vi "to string.vi"(8 "error in":errorcluster, 11 "Logic Sequencer configuration in":refnum<class "Logic Sequencer configuration.lvclass">) -> (0 "error out":errorcluster, 1 "data":string, 2 "version":string, 3 "Logic Sequencer configuration out":refnum<class "Logic Sequencer configuration.lvclass">)   [LabVIEW 2013, in "Logic Sequencer configuration.lvclass"]
doc: "Provides an interface for saving a module configuration to a file or other serialized data source. It is recommended that all children of this class store data in two sets--data required for its own initialization, and any data required for parent initialization--and that each implementation uses the <b>Call Parent Method</b> primitive to serialize parent information."
uses:
  Logic Sequencer configuration.lvclass
  <vilib>/NI/Tag Bus Module Framework/module configuration/TBM module configuration.lvclass
  Logic Sequencer configuration.lvclass/Logic Sequencer configuration.ctl
  <vilib>/NI/Tag Bus Module Framework/root configuration/unwrap data.vi
  current version.vi
  <vilib>/NI/Tag Bus Module Framework/root configuration/TBM configuration.lvclass
  <vilib>/NI/Tag Bus Module Framework/channel/TBM channel.lvclass
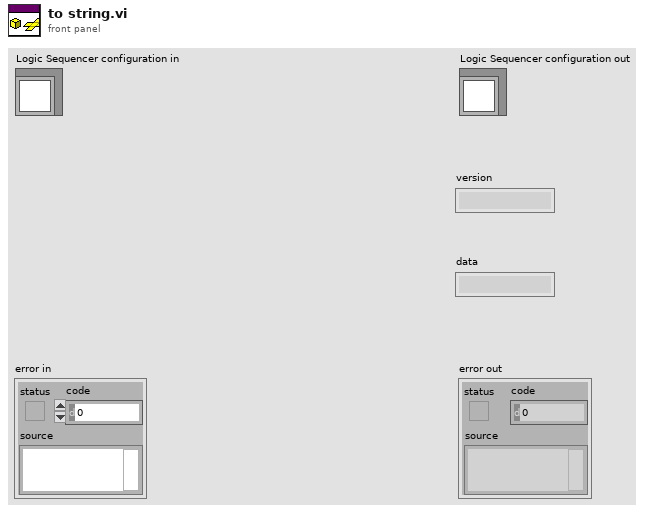
[diagram p1: front panel]
types:
  T1 = typedef "Logic Sequencer configuration.lvclass/processing channels.ctl" = cluster{"parameter":refnum<class "TBM channel.lvclass">, "result":refnum<class "TBM channel.lvclass">}
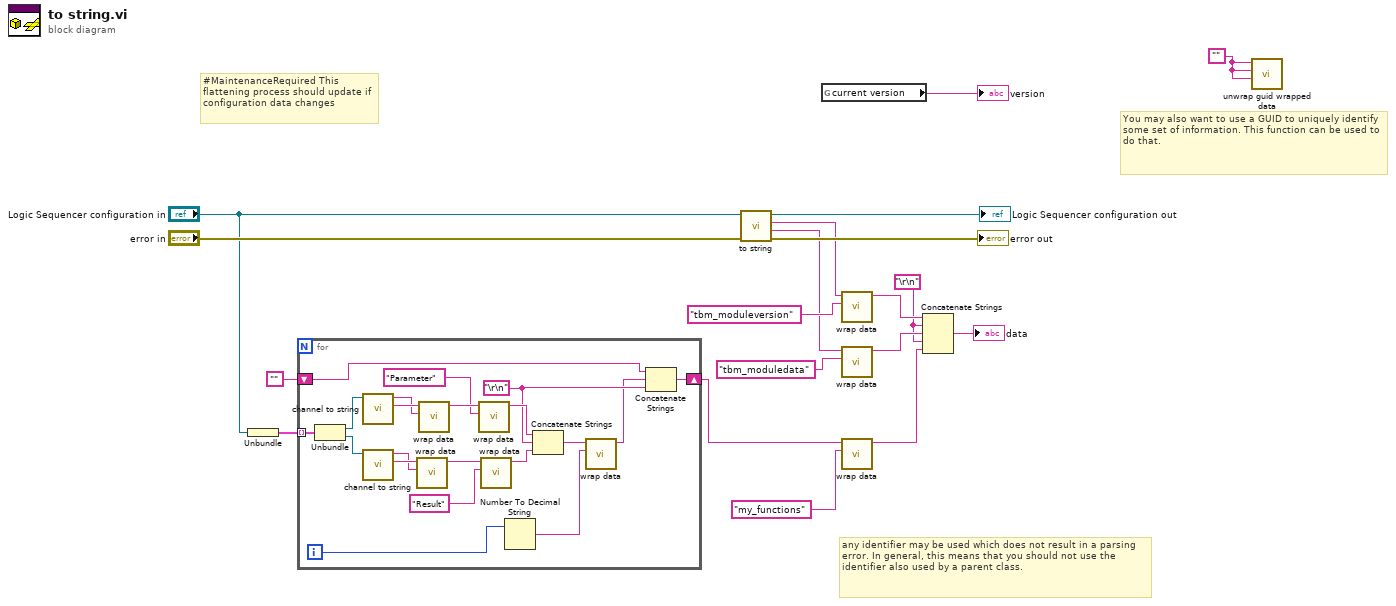
[diagram p0: block diagram]
diagram:
  w1 = "\r\n"
  w11 = ""
  # "any identifier may be used which does not result in a parsing error. In general, this means that you should not use the identifier also used by a parent class."
  # "You may also want to use a GUID to uniquely identify some set of information. This function can be used to do that."
  # "#MaintenanceRequired This flattening process should update if configuration data changes"
  n1 = Unbundle("Logic Sequencer configuration in") -> (w5:T1[])
  n2 = for {
    tunnel: w5 -> [w39] mode=indexing
    shift-right: [w26] -> w3
    shift-left: "" -> [w25]
    i -> [w23]
    w24 = "\r\n"
    n3 = Unbundle(w39) -> ("parameter"=w38:refnum<class "TBM channel.lvclass">, "result"=w37:refnum<class "TBM channel.lvclass">)
    n4 = call <vilib>:"channel to string.vi"("channel in"=w38) -> ("channel data"=w36:string, "identifier"=w33:string)  [unwired: 9 in]
    n5 = call <vilib>:"channel to string.vi"("channel in"=w37) -> ("channel data"=w35:string, "identifier"=w34:string)  [unwired: 9 in]
    n6 = call <vilib>:"wrap data.vi"("identifier"=w34, "data to wrap"=w35) -> ("wrapped data"=w30:string)  [unwired: 9 in]
    n7 = call <vilib>:"wrap data.vi"("identifier"=w33, "data to wrap"=w36) -> ("wrapped data"=w32:string)  [unwired: 9 in]
    n8 = call <vilib>:"wrap data.vi"("identifier"="Parameter", "data to wrap"=w32) -> ("wrapped data"=w28:string)  [unwired: 9 in]
    n9 = call <vilib>:"wrap data.vi"("identifier"="Result", "data to wrap"=w30) -> ("wrapped data"=w27:string)  [unwired: 9 in]
    n10 = Number To Decimal String(number=w23) -> (decimal integer string=w21:string)  [unwired: 1 in]
    n11 = Concatenate Strings(w28, w24, w27) -> (w22:string)
    n12 = call <vilib>:"wrap data.vi"("identifier"=w21, "data to wrap"=w22) -> ("wrapped data"=w20:string)  [unwired: 9 in]
    n13 = Concatenate Strings(w25, w20, w24) -> (w26:string)
  }
  n14 = call-parent "to string.vi"("error in"="error in", "module configuration in"="Logic Sequencer configuration in") -> ("error out"=→"error out":errorcluster, "data"=w6:string, "version"=w7:string, "module configuration out"=→"Logic Sequencer configuration out":refnum<class "Logic Sequencer configuration.lvclass">)  [unwired: 6 in]
  n15 = global read "current version.vi" "current version"() -> (→"version":string)
  n16 = call <vilib>:"wrap data.vi"("identifier"="tbm_moduleversion" ("additional identifier"), "data to wrap"=w7) -> ("wrapped data"=w13:string)  [unwired: 9 in]
  n17 = call <vilib>:"wrap data.vi"("identifier"="tbm_moduledata" ("additional identifier"), "data to wrap"=w6) -> ("wrapped data"=w12:string)  [unwired: 9 in]
  n18 = call <vilib>:"wrap data.vi"("identifier"="my_functions" ("additional identifier"), "data to wrap"=w3) -> ("wrapped data"=w2:string)  [unwired: 9 in]
  n19 = Concatenate Strings(w13, w1, w12, w1, w2) -> (→"data":string)
  n20 = call <vilib>:"unwrap guid wrapped data.vi"("identifier"=w11, "uuid"=w11, "data to unwrap"=w11) -> ()  [unwired: 7 in, 2 out]
